vi "Finish.vi"(8 "error in (no error)":errorcluster, 11 "Comp Trace Logger in":refnum<class "Comp Trace Logger.lvclass">) -> (0 "error out":errorcluster, 3 "Comp Trace Logger out":refnum<class "Comp Trace Logger.lvclass">)   [LabVIEW 2014, in "Comp Trace Logger.lvlib" / "Comp Trace Logger.lvclass"]
uses:
  Comp Trace Logger.lvclass
  Comp Trace Logger.lvclass/Comp Trace Logger.ctl
  Robot Actor Framework/Trace/Trace Listener Class/Trace Listener.lvclass
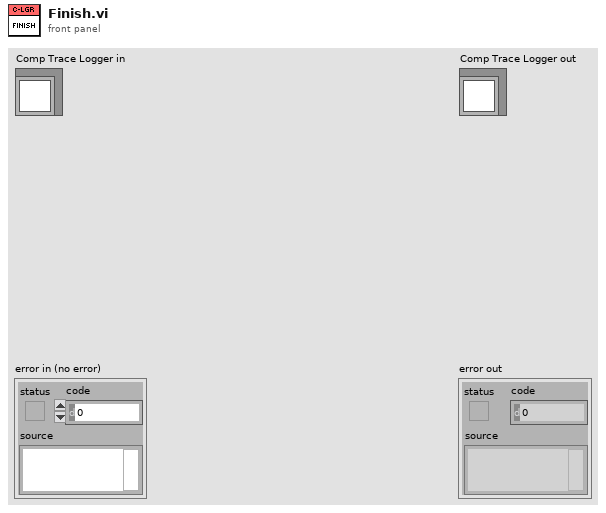
[diagram p1: front panel]
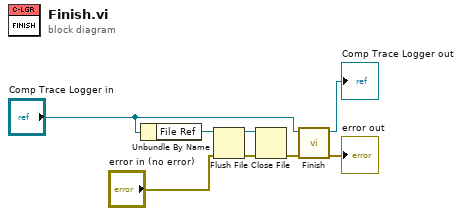
[diagram p0: block diagram]
diagram:
  n1 = Unbundle By Name("Comp Trace Logger in") -> ("File Ref"=w5:refnum<file>)
  n2 = Flush File(refnum=w5, error in="error in (no error)") -> (refnum out=w4:refnum<file>, error out=w2:errorcluster)
  n3 = Close File(refnum=w4, error in=w2) -> (error out=w1:errorcluster)  [unwired: 1 out]
  n4 = call-parent "Finish.vi"("error in (no error)"=w1, "System Actor in"="Comp Trace Logger in") -> ("error out"=→"error out":errorcluster, "System Actor out"=→"Comp Trace Logger out":refnum<class "Comp Trace Logger.lvclass">)  [unwired: 8 in]
